vi "Decompose Command String.vi"(8 "Error In":errorcluster, 11 "Command IN":string) -> (0 "Error Out":errorcluster, 1 "Parameter Text":string, 2 "Parameter Table":string[][](array[string]), 3 "Action":string)   [LabVIEW 2012]
doc: "SciScan 1.2 160622"
uses:
  <vilib>/regexp/Match Regular Expression.xnode
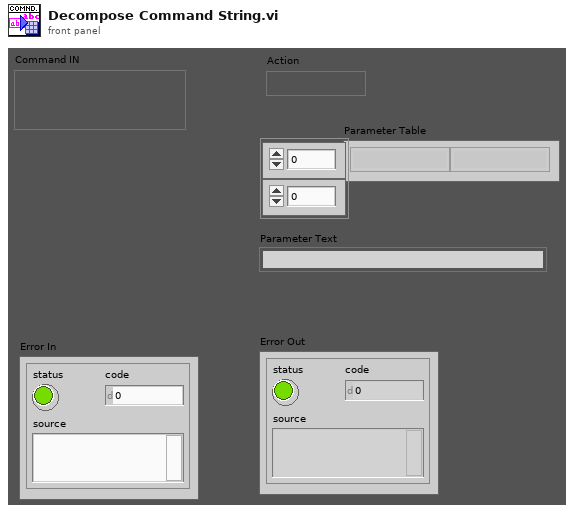
[diagram p1: front panel]
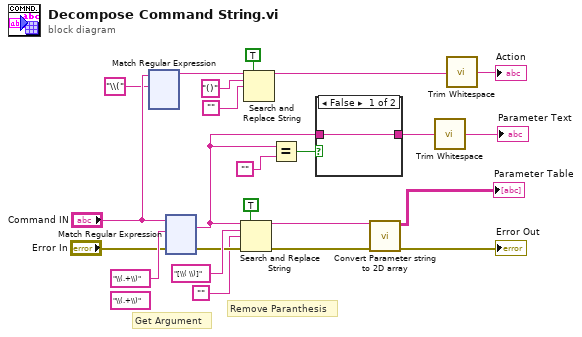
[diagram p0: block diagram]
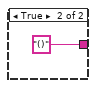
[diagram p2: hidden frame]
diagram:
  (unwired) "\\(.+\\)" ("search string/char (-)")
  # "Get Argument"
  # "Remove Paranthesis"
  n1 = xnode "Match Regular Expression"("input string"="Command IN", "regular expression"="\\(") -> ("before match"=w12:string)  [unwired: 4 in, 4 out]
  n2 = xnode "Match Regular Expression"("input string"="Command IN", "regular expression"="\\(.+\\)" ("search string/char (-)"), "error in"="Error In") -> ("whole match"=w5:string, "error out"=w21:errorcluster)  [unwired: 3 in, 3 out]
  n3 = Search and Replace String(replace all?=TRUE ("replace all? (F)"), input string=w5, search string="[\\( \\)]", replace string="", error in=w21) -> (result string=w11:string, error out=w10:errorcluster)  [unwired: 3 in, 2 out]
  n4 = Search and Replace String(replace all?=TRUE ("replace all? (F)"), input string=w12, search string="()", replace string="") -> (result string=w3:string)  [unwired: 4 in, 3 out]
  n5 = Equal?(x=w5, y="") -> (x = y?=w6:bool)
  n6 = case shown="False" w6 {
    tunnel: w5 -> [w24 _]
    tunnel: [w24 "()" ("search string/char (-)")] -> w2
    frame False {
    }
    frame True {
    }
  }
  n7 = call "Convert Parameter string to 2D array.vi"("Error In"=w10, "Parameter string IN (without paranthesis)"=w11) -> ("Error Out"=→"Error Out":errorcluster, "Params table OUT"=→"Parameter Table":string[][])  [unwired: 6 in, 2 out]
  n8 = call <vilib>:"Trim Whitespace.vi"("string"=w2) -> ("trimmed string"=→"Parameter Text":string)  [unwired: 1 in]
  n9 = call <vilib>:"Trim Whitespace.vi"("string"=w3) -> ("trimmed string"=→"Action":string)  [unwired: 1 in]
